vi "Arduino_6_0.vi"() -> ()   [LabVIEW 2015]
uses:
  <vilib>/LabVIEW Interface for Arduino/LabVIEW Interface for Arduino.lvlib
panel:
  in  "PIR 2":u8
  out "LED OFF when Room is empty":bool
  out "Total":i32
  out "person exit Room PIR_2":i32
  out "PIR 2":dbl(knob) scale=0.0..5.0
  out "person in Room PIR_1":i32
  in  "PIR 1":u8
  out "PIR":dbl(knob) scale=0.0..5.0
  in  "stop":bool
  in  "VISA resource":refnum<visa-resource-name>
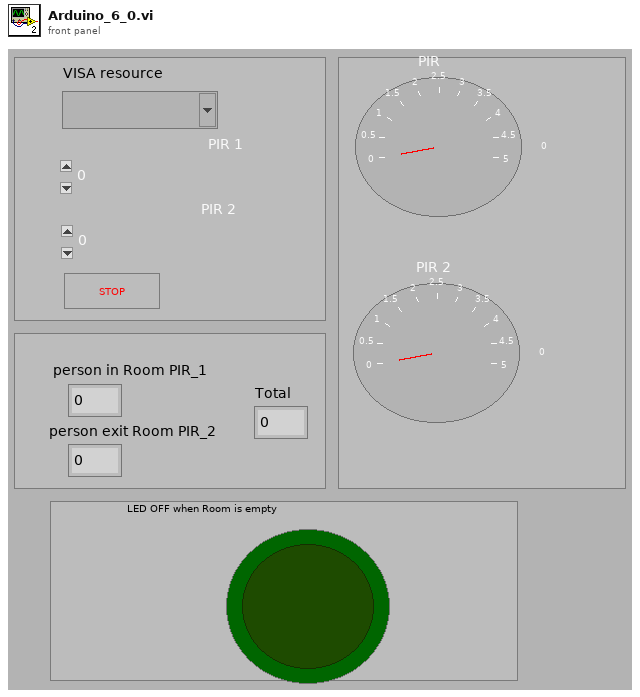
[diagram p1: front panel]
types:
  T1 = typedef "LabVIEW Interface for Arduino.lvlib/Arduino Resource.ctl" = cluster{"VISA resource":refnum<visa-resource-name>, "Board Type":T2, "Connection Type":enum8{"USB / Serial"}, "Bytes Per Packet (15)":u8}
  T2 = typedef "LabVIEW Interface for Arduino.lvlib/Board Type.ctl" = enum16{"Uno", "Dimuelanove w/Atmega 328", "Mega 2560"}
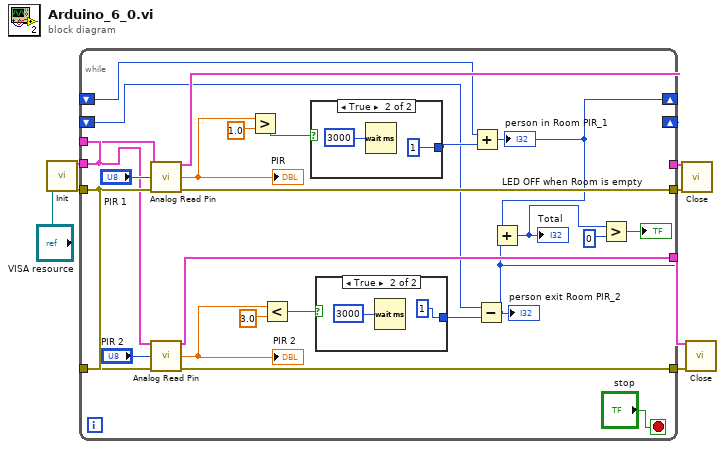
[diagram p0: block diagram]
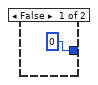
[diagram p2: hidden frame]
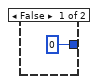
[diagram p3: hidden frame]
diagram:
  n1 = call <vilib>:"Init.vi"("VISA resource"="VISA resource") -> ("Arduino Resource"=w4:T1, "error out"=w3:errorcluster)  [unwired: 17 in]
  n2 = while {
    tunnel: w4 -> [w30]
    tunnel: [w33] -> w7
    tunnel: [w32] -> w6
    tunnel: w3 -> [w29]
    shift-right: [w13] -> _
    shift-left: _ -> [w25]
    tunnel: w4 -> [w22]
    tunnel: w3 -> [w21]
    tunnel: [w20] -> w2
    tunnel: [w19] -> w1
    shift-right: [w12] -> _
    shift-left: _ -> [w15]
    stop <- "stop" stop-if-true
    n3 = call <vilib>:"Analog Read Pin.vi"("Arduino Resource"=w30, "Analog Input Pin (0)"="PIR 1", "error in"=w29) -> ("Arduino Resource"=w33:T1, "Voltage"=w23:dbl, "error out"=w32:errorcluster)  [unwired: 10 in]
    "PIR" <- w23
    n4 = call <vilib>:"Analog Read Pin.vi"("Arduino Resource"=w22, "Analog Input Pin (0)"="PIR 2", "error in"=w21) -> ("Arduino Resource"=w20:T1, "Voltage"=w17:dbl, "error out"=w19:errorcluster)  [unwired: 10 in]
    "PIR 2" <- w17
    n5 = Greater?(x=w23, y=1.0) -> (0:w26:bool)
    n6 = Less?(x=w17, y=3.0) -> (x < y?=w18:bool)
    n7 = case shown="True" w26 {
      tunnel: [0 1] -> w24
      frame False {
      }
      frame True {
        n8 = Wait (ms)(milliseconds to wait=u32 3000) -> ()  [unwired: 1 out]
      }
    }
    n9 = case shown="True" w18 {
      tunnel: [0 1] -> w14
      frame False {
      }
      frame True {
        n10 = Wait (ms)(milliseconds to wait=u32 3000) -> ()  [unwired: 1 out]
      }
    }
    n11 = Add(x=w25, y=w24) -> (x+y=w13:i32)
    "person in Room PIR_1" <- w13
    n12 = Subtract(x=w15, y=w14) -> (x-y=w12:i32)
    "person exit Room PIR_2" <- w12
    n13 = Add(x=w13, y=w12) -> (x+y=w10:i32)
    "Total" <- w10
    n14 = Greater?(x=w10, y=0) -> (0:→"LED OFF when Room is empty":bool)
  }
  n15 = call <vilib>:"Close.vi"("Arduino Resource"=w7, "error in"=w6) -> ()  [unwired: 13 in, 1 out]
  n16 = call <vilib>:"Close.vi"("Arduino Resource"=w2, "error in"=w1) -> ()  [unwired: 13 in, 1 out]
